vi "Specify Delete Action.vi"(11 "ARN in":refnum<class "ARN.lvclass">) -> (2 "Delete action":string, 3 "ARN out":refnum<class "ARN.lvclass">)   [LabVIEW 2015, in "NI_AWS_Core.lvlib" / "ARN.lvclass"]
uses:
  ARN.lvclass
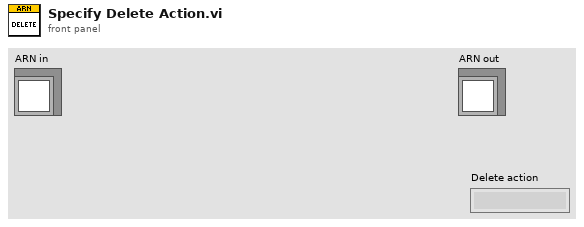
[diagram p1: front panel]
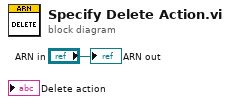
[diagram p0: block diagram]
diagram:
  "ARN out" <- "ARN in"
